vi "DFD Filtering (PtByPt).vi"(7 "init? (F)":bool, 8 "error in (no error)":errorcluster, 10 "filter":T1={"mSRate_Fs"=1.0, "mSRate_Version"="2.0", "mSRate_Comments"="", "mSRate_OrgCoef"={"type"=enum."Undefined", "gain"=1.0, "coef a (k)"=[], "coef b (v)"=[]}, "mSRate_CurCoef"={"type"=enum."Undefined", "gain"=1.0, "coef a (k)"=[], "coef b (v)"=[]}, "mSRate_Quantized?"=FALSE, "mSRate_QCoef"={"type"=enum."Undefined", "gain"=1.0, "coef a (k)"=[], "coef b (v)"=[]}, "mSRate_QSettings"=[], "mSRate_Order"=0, "mSRate_Scaling"={"mSRate_ScaleByPowerOf2?"=FALSE, "mSRate_ScaleType"=enum."No Norm"}} {"mSRate_QSettings"."source" items=["Coef a/k"=0, "Coef b/v"=7, "Input"=1, "Output"=2, "Multiplicand"=3, "Product"=4, "Sum"=5, "Delay"=6, "Gain"=8]}, 11 "signal in":dbl) -> (0 "error out":errorcluster, 3 "signal out":dbl)   [LabVIEW 2017, in "NI_DigFilterLicensed.lvlib"]
doc: "Filters an input signal continuously. Wire data to the <B>signal in</B> input to determine the polymorphic instance to use or manually select the instance."
uses:
  <vilib>/addons/Digital Filter Design/NI_DigFilterLicensed.lvlib
  <vilib>/addons/Digital Filter Design/_Objects.llb/DFD Filter Obj.ctl
  <vilib>/addons/Digital Filter Design/_Objects.llb/DFD Filter Coef.ctl
  <vilib>/addons/Digital Filter Design/_Objects.llb/DFD Filter Structure Type Selector.ctl
  <vilib>/addons/Digital Filter Design/_Objects.llb/dfd_Internal Quantization Settings.ctl
  <vilib>/addons/Digital Filter Design/_Objects.llb/dfd_Internal Quantization Srcs.ctl
  <vilib>/addons/Digital Filter Design/_Objects.llb/DFD Coef Norm Type.ctl
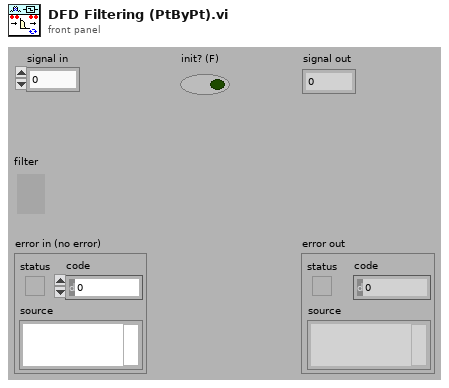
[diagram p1: front panel]
types:
  T1 = typedef "NI_DigFilterLicensed.lvlib/DFD Filter Obj.ctl" = cluster{"mSRate_Fs":dbl, "mSRate_Version":string, "mSRate_Comments":string, "mSRate_OrgCoef":T2, "mSRate_CurCoef":T2, "mSRate_Quantized?":bool, "mSRate_QCoef":T2, "mSRate_QSettings":T4[], "mSRate_Order":i32, "mSRate_Scaling":cluster{"mSRate_ScaleByPowerOf2?":bool, "mSRate_ScaleType":T6}}
  T2 = typedef "NI_DigFilterLicensed.lvlib/DFD Filter Coef.ctl" = cluster{"type":T3, "gain":dbl, "coef a (k)":dbl[], "coef b (v)":dbl[]}
  T3 = typedef "NI_DigFilterLicensed.lvlib/DFD Filter Structure Type Selector.ctl" = enum16{"Undefined", "FIR Direct Form", "FIR Direct Form Transposed", "FIR Symmetric", "FIR Antisymmetric", "IIR Direct Form I", "IIR Direct Form I Transposed", "IIR Direct Form II", "IIR Direct Form II Transposed", "IIR Cascaded Second Order Sections Form I", "IIR Cascaded Second Order Sections Form I Transposed", "IIR Cascaded Second Order Sections Form II", "IIR Cascaded Second Order Sections Form II Transposed", "Lattice Allpass (basic sections)", "Lattice Allpass (one multiplier sections)", "Lattice Allpass (normalized sections)", "Lattice AR (basic sections)", "Lattice AR (one multiplier sections)", "Lattice AR (normalized sections)", "Lattice MA (minimum phase)", "Lattice MA (maximum phase)", "Lattice ARMA (basic sections)", "Lattice ARMA (one multiplier sections)", "Lattice ARMA (normalized sections)"}
  T4 = typedef "NI_DigFilterLicensed.lvlib/dfd_Internal Quantization Settings.ctl" = cluster{"source":T5, "wl":i16, "iwl":i16, "overflow mode":enum16{"Saturation", "Wrap"}, "rounding mode":enum16{"Nearest", "Truncation"}, "signed?":bool}
  T5 = typedef "NI_DigFilterLicensed.lvlib/dfd_Internal Quantization Srcs.ctl" = u16
  T6 = typedef "NI_DigFilterLicensed.lvlib/DFD Coef Norm Type.ctl" = enum16{"No Norm", "Time Domain 1-Norm", "Time Domain 2-Norm", "Time Domain Inf-Norm"}
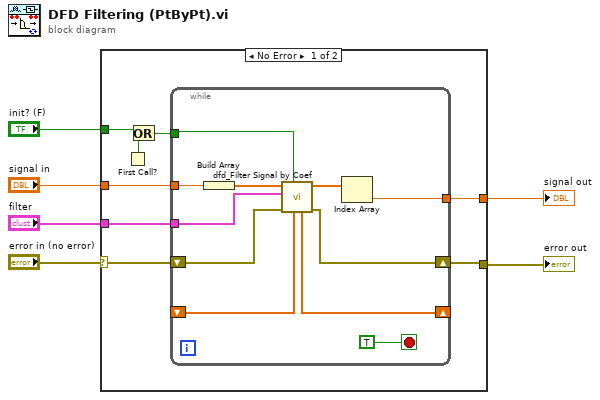
[diagram p0: block diagram]
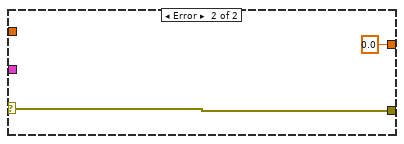
[diagram p2: hidden frame]
diagram:
  n1 = case shown="No Error" "error in (no error)" {
    selector: "error in (no error)" -> [w12 w27]
    tunnel: [w7 w27] -> w5
    tunnel: "filter" -> [w13 _]
    tunnel: "signal in" -> [w14 _]
    tunnel: [w8 0.0 ("number: 0 to 1")] -> w2
    tunnel: "init? (F)" -> [w10 _]
    frame No Error {
      n2 = First Call?() -> (First Call?: T/F=w11:bool)
      n3 = Or(x=w10, y=w11) -> (x .or. y?=w9:bool)
      n4 = while {
        tunnel: w14 -> [w24]
        tunnel: w13 -> [w21]
        shift-right: [w17] -> _
        shift-left: _ -> [w18]
        tunnel: w9 -> [w22]
        tunnel: [w19] -> w8
        shift-right: [w15] -> w7
        shift-left: w12 -> [w16]
        stop <- TRUE stop-if-true
        n5 = Build Array(w24) -> (w23:dbl[])
        n6 = call <vilib>:"dfd_Filter Signal by Coef.vi"("state in"=w18, "initH?"=w22, "error in(no error)"=w16, "filter"=w21, "x"=w23) -> ("error out"=w15:errorcluster, "filtered x"=w20:dbl[], "state out"=w17:dbl[])  [unwired: 1 in, 3 out]
        n7 = Index Array(array=w20) -> (element=w19:dbl)  [unwired: 1 in]
      }
    }
    frame Error {
    }
  }
  "error out" <- w5
  "signal out" <- w2
